vi "omega reading-working.vi"() -> ()   [LabVIEW 2010]
uses:
  <vilib>/Instr/_visa.llb/VISA Configure Serial Port (Instr).vi
panel:
  in  "stop":bool
  in  "VISA Omega (Serial - COM1)":refnum<visa-resource-name>="COM1"
  out "value":dbl
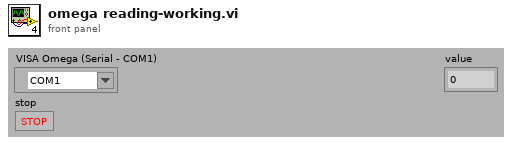
[diagram p1: front panel]
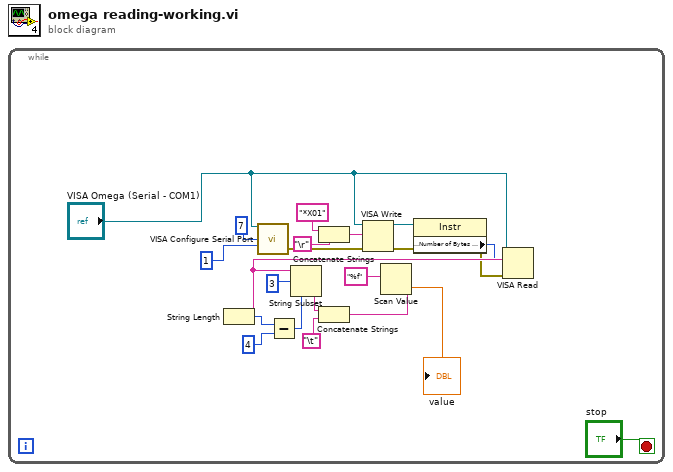
[diagram p0: block diagram]
diagram:
  n1 = while {
    stop <- "stop" stop-if-true
    n2 = call-poly "VISA Configure Serial Port"("VISA resource name"="VISA Omega (Serial - COM1)", "data bits (8)"=7, "parity (0:none)"=1) -> ("error out"=w8:errorcluster)  [unwired: 11 in, 1 out]
    n3 = Concatenate Strings("*X01", "\r") -> (w11:string)
    n4 = VISA Write(VISA resource name="VISA Omega (Serial - COM1)", write buffer=w11, error in (no error)=w8) -> (VISA resource name out=w22:refnum<visa-resource-name>, error out=w12:errorcluster)  [unwired: 1 out]
    n5 = property class="Instr"(reference=w22, error in=w12) -> (error out=w13:errorcluster, "Serial Settings:Number of Bytes at Serial Port"=w14:u32)  [unwired: 1 out]
    n6 = VISA Read(VISA resource name="VISA Omega (Serial - COM1)", byte count=w14, error in (no error)=w13) -> (read buffer=w15:string)  [unwired: 3 out]
    n7 = String Length(string=w15) -> (length=w17:i32)
    n8 = Subtract(x=w17, y=4) -> (x-y=w19:i32)
    n9 = String Subset(string=w15, offset (0)=3, length (rest)=w19) -> (substring=w20:string)
    n10 = Concatenate Strings(w20, "\t") -> (w4:string)
    n11 = Scan Value(string=w4, format string="%f") -> (value=→"value":dbl)  [unwired: 1 in, 1 out]
  }
